vi "UPD Variable Init.vi"(11 "Expt Name":string) -> (0 "Mcast Address":string, 1 "UDP timeout ms":i32=2000, 2 "MC Multicast":refnum<k16>, 3 "My IP":string, 4 "Mcast remote":u16, 6 "> Name, devtype, ip, dev comm port, class, location for all devices>":string[][](array[string]))   [LabVIEW 2020]
uses:
  Shared/MySQL/Preset Query Enum.ctl
  <vilib>/Utility/tcp.llb/UDP Multicast Write-Only Open.vi
panel:
  out "error out":errorcluster
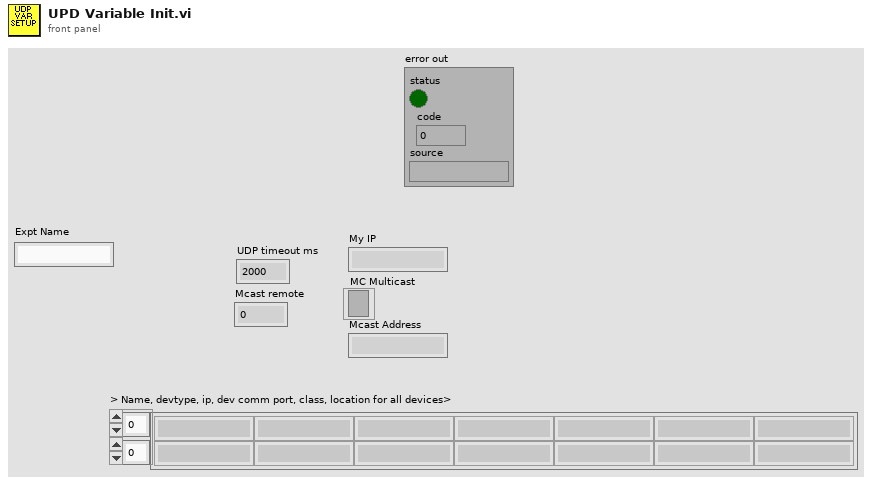
[diagram p1: front panel]
types:
  T1 = typedef "Preset Query Enum.ctl" = enum16{"Get Locations", "Get all IPs and MACs", "Get classes", "Get expt variables to set at scanstart for particular device", "Get expt devices and variables with start values", "Get expt devices and variables (with data to get)", "Get expt devices with data to get", "Get Expt devices and GUIs", "Get all devices basic properties", "Get Virtual Devices Core Info", "Get Expt names", "Get experiment basic properties", "Get experiment alarm variables", "Get MC Ports", "Get device network comm port", "Get devicetype lvclass path", "Get basic device properties", "Get Init Order", "Get all setable variables of a device", "Get device variable aliases", "Get force values of all settable variables", "Get all variables of a devicetype", "Get all variables of a device", "Get plotter details", "Get Saved Scans", "Get Scan Info", "GetGeneralGUIs", "Get expt for plotter", "Get plotter IDs from expt", "Get all devices", "Get all Virtual Devices", "Get all aliases", "Get variable and device info for Virtual Device", "GetItemLocatorIP", "Get IPs for GUIs", "Get DeviceType from Device", "GetLocalPortRange", "GetDevicePresetVariables", "Get Device Configuration", "GetAllPresetNames", "GetAllConfigurationNames", "GetPresetDeviceNames", "GetDeviceAliases", "GetDevicesOfClass"}
  T2 = typedef "MCports.ctl" = cluster{"Mcast local":u16, "Mcast remote":u16, "udp local":u16, "udp local slow":u16, "udp lvstarter":u16}
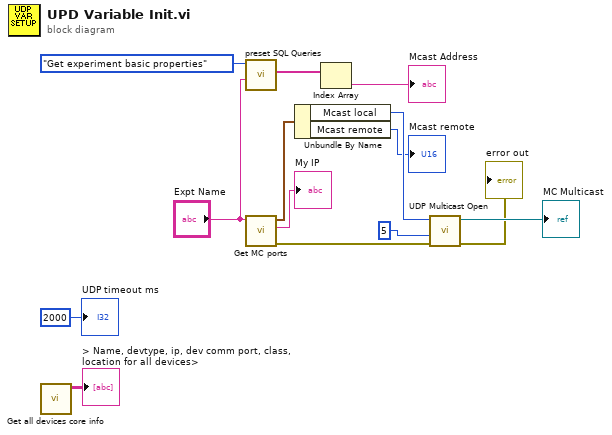
[diagram p0: block diagram]
diagram:
  n1 = call "Get all devices core info.vi"() -> ("> Name, devtype, ip, dev comm port, class, location for all devices>"=→"> Name, devtype, ip, dev comm port, class, location for all devices>":string[][])  [unwired: 8 in, 3 out]
  n2 = call "preset SQL Queries.vi"("Expt name / MCIP/ Variable/Preset Name"="Expt Name", "Preset Query"=Preset_Query_Enum."Get experiment basic properties") -> ("1st column 1st data"=w6:string[])  [unwired: 7 in, 2 out]
  n3 = call "Get MC ports.vi"("Expt name / MCIP/ Variable Name"="Expt Name") -> ("error out"=w14:errorcluster, "IP"=→"My IP":string, "MC Port Cluster"=w12:T2)  [unwired: 8 in]
  n4 = Unbundle By Name(w12) -> ("Mcast local"=w13:u16, "Mcast remote"=→"Mcast remote":u16)
  n5 = Index Array(array=w6) -> (element=→"Mcast Address":string)  [unwired: 1 in]
  n6 = call-poly <vilib>:"UDP Multicast Open.vi"("error in (no error)"=w14, "time-to-live (1)"=u16 5, "port"=w13) -> ("error out"=→"error out":errorcluster, "connection ID"=→"MC Multicast":refnum<k16>)  [unwired: 7 in]
  "UDP timeout ms" <- 2000 ("Preset Manager Cluster.UDP timeout ms")
